vi "load_validation_file.vi"(6 "LUA Validation File":path, 10 "Parameters Tree":refnum<vi>) -> (2 "Vali File Loaded":bool, 3 "# Lines":i32)   [LabVIEW 2019]
uses:
  Biogas_LabView_Wrapper/lib/libBioGasLabViewWrapper.so
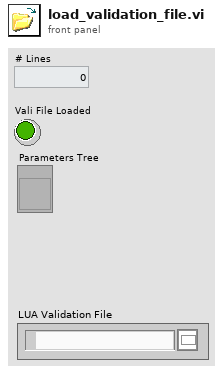
[diagram p1: front panel]
types:
  T1 = cluster{string, string[], "Child Tag":string, i32, "Child Only?":bool, i32}
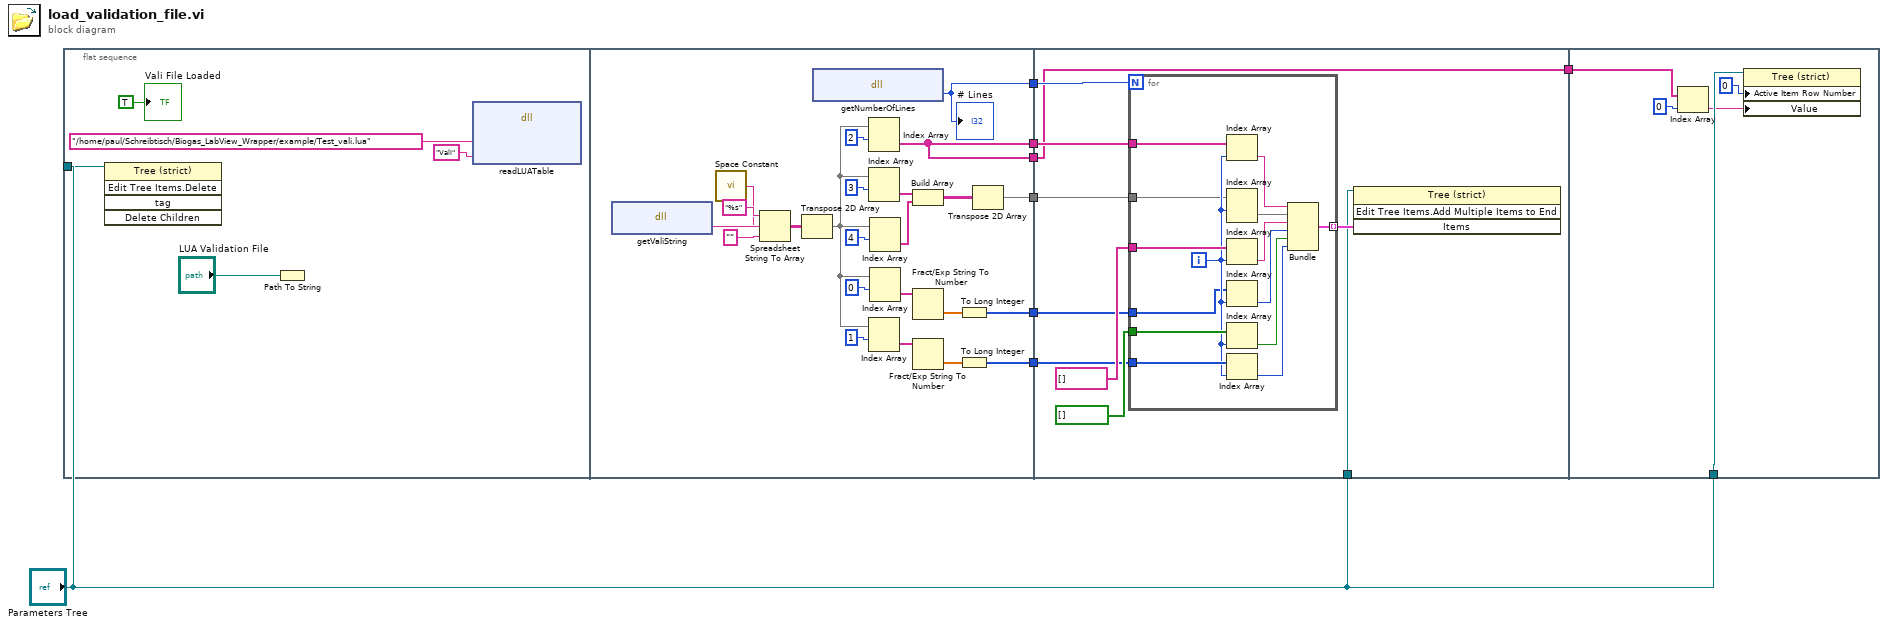
[diagram p0: block diagram]
diagram:
  n1 = flat-sequence {
    tunnel: "Parameters Tree" -> [w9]
    tunnel: [w32] -> w8
    tunnel: [w27] -> w6
    tunnel: [w23] -> w5
    tunnel: [w16] -> w4
    tunnel: [w16] -> w2
    tunnel: [w14] -> w1
    tunnel: w8 -> [w43]
    tunnel: "Parameters Tree" -> [w42]
    tunnel: w6 -> [w41]
    tunnel: w5 -> [w40]
    tunnel: w4 -> [w39]
    tunnel: [w38] -> w3
    tunnel: w2 -> [w38]
    tunnel: w1 -> [w37]
    tunnel: "Parameters Tree" -> [w63]
    tunnel: w3 -> [w62]
    frame #0 {
      n2 = invoke on="Invoke Node" class="Tree (strict)" method="Edit Tree Items.Delete"(reference=w9) -> ()  [unwired: 4 in, 5 out]
      n3 = Path To String(path="LUA Validation File") -> ()  [unwired: 1 out]
      n4 = dll-call lib="home/paul/Schreibtisch/Biogas_LabView_Wrapper/lib/libBioGasLabViewWrapper.so" fn="readLUATable"("filename"="/home/paul/Schreibtisch/Biogas_LabView_Wrapper/example/Test_vali.lua", "vali_or_spec"="Vali" ("spec_filename")) -> ()  [unwired: 6 in, 2 out]
      "Vali File Loaded" <- TRUE ("Vali File Loaded")
    }
    frame #1 {
      n5 = dll-call lib="home/paul/Schreibtisch/Biogas_LabView_Wrapper/lib/libBioGasLabViewWrapper.so" fn="getValiString"() -> ("return type"=w36:string)  [unwired: 3 in, 2 out]
      n6 = call <vilib>:"Space Constant.vi"() -> ("String"=w31:string)
      n7 = Spreadsheet String To Array(delimiter (Tab)=w31, format string="%s", spreadsheet string=w36, array type (2D Dbl)="") -> (array=w33:string[][])
      n8 = Transpose 2D Array(2D array=w33) -> (transposed array=w20:string[][])
      n9 = dll-call lib="home/paul/Schreibtisch/Biogas_LabView_Wrapper/lib/libBioGasLabViewWrapper.so" fn="getNumberOfLines"() -> ("numLines"=w32:i32)  [unwired: 3 in, 2 out]
      "# Lines" <- w32
      n10 = Index Array(array=w20, index (row)=2) -> (element=w16:string[])  [unwired: 1 in]
      n11 = Index Array(array=w20, index (row)=3) -> (element=w18:string[])  [unwired: 1 in]
      n12 = Index Array(array=w20, index (row)=1) -> (element=w25:string[])  [unwired: 1 in]
      n13 = Index Array(array=w20, index (row)=4) -> (element=w17:string[])  [unwired: 1 in]
      n14 = Index Array(array=w20, index (row)=0) -> (element=w29:string[])  [unwired: 1 in]
      n15 = Build Array(w18, w17) -> (w15:string[][])
      n16 = Fract/Exp String To Number(string=w29) -> (number=w28:dbl[])  [unwired: 3 in, 1 out]
      n17 = Fract/Exp String To Number(string=w25) -> (number=w24:dbl[])  [unwired: 3 in, 1 out]
      n18 = To Long Integer(number=w28) -> (32bit integer=w27:i32[])
      n19 = To Long Integer(number=w24) -> (32bit integer=w23:i32[])
      n20 = Transpose 2D Array(2D array=w15) -> (transposed array=w14:string[][])
    }
    frame #2 {
      n21 = for {
        N: w43 -> [_]
        tunnel: w39 -> [w60]
        tunnel: string[] [] ("Child Tag") -> [w59]
        tunnel: w41 -> [w47]
        tunnel: bool[] [] ("Child Only?") -> [w58]
        tunnel: w40 -> [w57]
        tunnel: [w51] -> w46 mode=indexing
        tunnel: w37 -> [w49]
        i -> [w50]
        n22 = Index Array(array=w60, index=w50) -> (element=w56:string)
        n23 = Index Array(array=w49, index (row)=w50) -> (element=w48:string[])  [unwired: 1 in]
        n24 = Index Array(array=w59, index=w50) -> (element=w55:string)
        n25 = Index Array(array=w47, index=w50) -> (element=w54:i32)
        n26 = Index Array(array=w58, index=w50) -> (element=w53:bool)
        n27 = Index Array(array=w57, index=w50) -> (element=w52:i32)
        n28 = Bundle(w56, w48, "Child Tag"=w55, w54, "Child Only?"=w53, w52) -> (w51:T1)  [unwired: 1 in]
      }
      n29 = invoke on="Invoke Node" class="Tree (strict)" method="Edit Tree Items.Add Multiple Items to End"(reference=w42, "Items"=w46) -> ()  [unwired: 2 in, 4 out]
    }
    frame #3 {
      n30 = Index Array(array=w62, index=0) -> (element=w61:string)
      n31 = property on="Property Node" class="Tree (strict)"(reference=w63, "Active Item Row Number"=0 ("Active Item:Row Number"), "Value"=w61) -> ()  [unwired: 1 in, 2 out]
    }
  }
